vi "Read Measurement Results.vi"(8 "error in":errorcluster, 11 "Instrument Driver in":refnum<class "Instrument Driver.lvclass">) -> (0 "error out":errorcluster, 2 "Measurement Results":T1={"Voltage (V)"=1.0} {"Voltage (V)" min=-424.2 max=424.2 step=1.0 format="%#.1f"}, 3 "Instrument Driver out":refnum<class "Instrument Driver.lvclass">)   [LabVIEW 2020, in "Plugin Instrument Driver.lvlib" / "Instrument Driver.lvclass"]
doc: "Read Measurement Results"
uses:
  Instrument Driver.lvclass
  Typedefs/Measurement Results.ctl
  Instrument Driver.lvclass/Instrument Driver.ctl
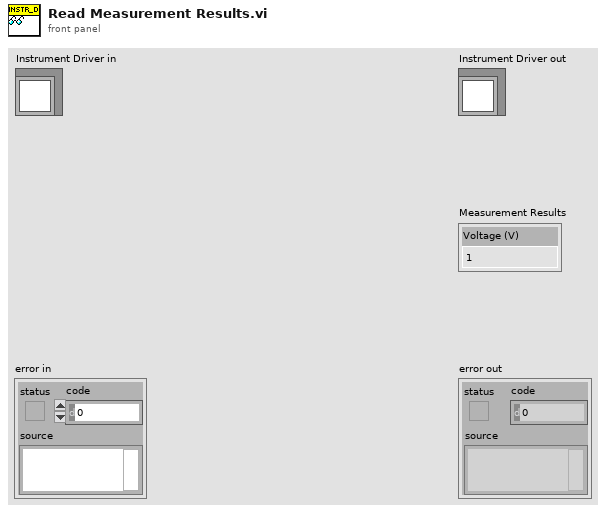
[diagram p1: front panel]
types:
  T1 = typedef "Plugin Instrument Driver.lvlib/Instrument Driver.lvclass/Measurement Results.ctl" = cluster{"Voltage (V)":dbl}
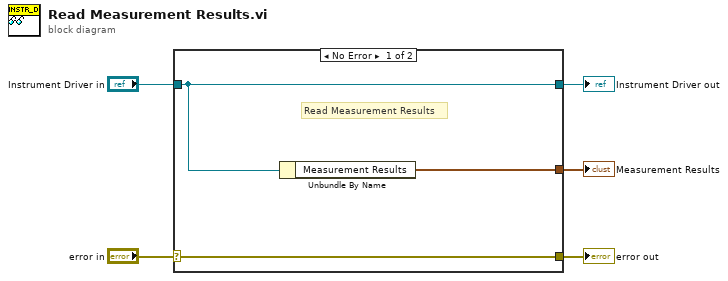
[diagram p0: block diagram]
diagram:
  n1 = case shown="No Error" "error in" {
    selector: "error in" -> [w8 w9]
    tunnel: [w8 w9] -> w4
    tunnel: [w7 w10] -> w2
    tunnel: "Instrument Driver in" -> [w7 w10]
    tunnel: [w6 _] -> w1
    frame No Error {
      # "Read Measurement Results"
      n2 = Unbundle By Name(w7) -> ("Measurement Results"=w6:T1)
    }
    frame Error {
    }
  }
  "error out" <- w4
  "Instrument Driver out" <- w2
  "Measurement Results" <- w1
